vi "Unpack Package.vi"(6 "Overwrite Target Directory if exists (TRUE)?":bool=TRUE, 8 "error in (no error)":errorcluster, 10 "Target directory (same as Package file if empty)":path, 11 "Package File":path) -> (0 "error out":errorcluster, 2 "Unpacked files":path[](array[path]), 3 "Unpacked Package Directory":path)   [LabVIEW 2020]
uses:
  <vilib>/zip/NI_Unzip.lvlib
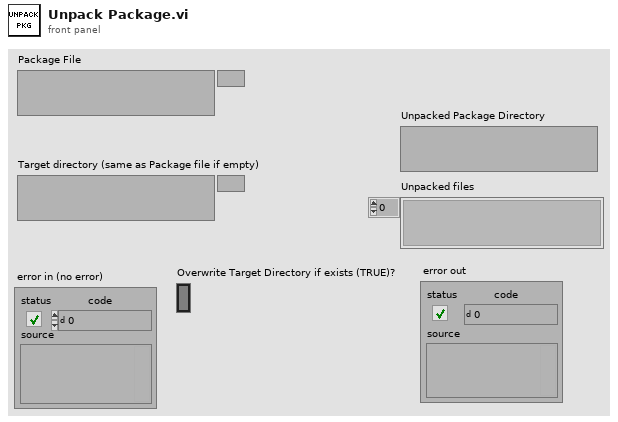
[diagram p1: front panel]
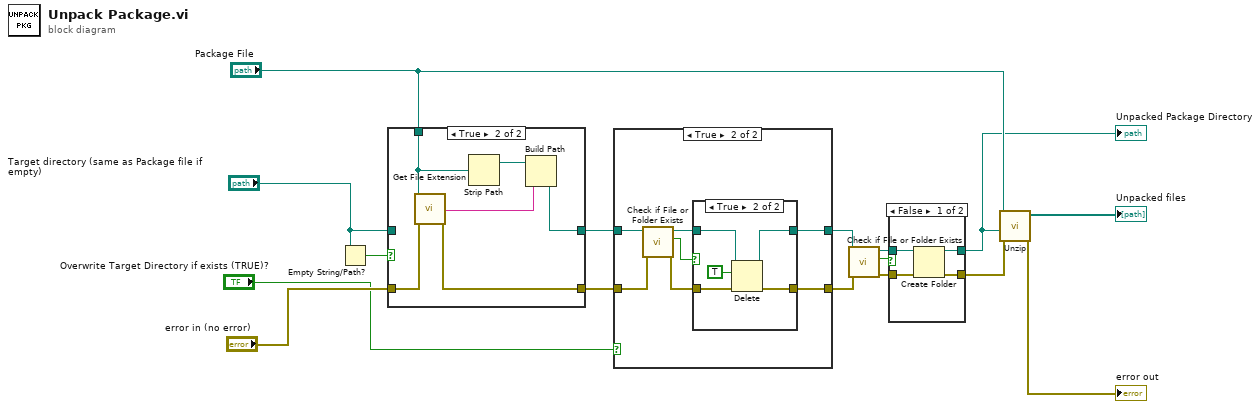
[diagram p0: block diagram]
diagram:
  n1 = Empty String/Path?(string/path="Target directory (same as Package file if empty)") -> (empty?=w16:bool)
  n2 = case shown="True" w16 {
    tunnel: "Package File" -> [_ w22]
    tunnel: "error in (no error)" -> [w18 w21]
    tunnel: [w18 w20] -> w13
    tunnel: [w17 w19] -> w12
    tunnel: "Target directory (same as Package file if empty)" -> [w17 _]
    frame False {
    }
    frame True {
      n3 = call <vilib>:"Get File Extension.vi"("error in (no error)"=w21, "file"=w22) -> ("error out"=w20:errorcluster, "filename without extension"=w23:string)  [unwired: 5 in, 3 out]
      n4 = Strip Path(path=w22) -> (stripped path=w24:path)  [unwired: 1 out]
      n5 = Build Path(base path=w24, name or relative path=w23) -> (appended path=w19:path)
    }
  }
  n6 = case shown="True" "Overwrite Target Directory if exists (TRUE)?" {
    tunnel: w13 -> [w25 w33]
    tunnel: w12 -> [w26 w32]
    tunnel: [w26 w28] -> w5
    tunnel: [w25 w27] -> w4
    frame False {
    }
    frame True {
      n7 = call <vilib>:"Check if File or Folder Exists.vi"("error in (no error)"=w33, "path"=w32) -> ("error out"=w30:errorcluster, "file or folder exists?"=w31:bool, "dup path"=w29:path)  [unwired: 7 in]
      n8 = case shown="True" w31 {
        tunnel: w30 -> [w35 w40]
        tunnel: w29 -> [w34 w38]
        tunnel: [w34 w37] -> w28
        tunnel: [w35 w36] -> w27
        frame False {
        }
        frame True {
          n9 = Delete(path (use dialog)=w38, entire hierarchy (F)=TRUE, error in=w40) -> (deleted path=w37:path, error out=w36:errorcluster)  [unwired: 2 in, 1 out]
        }
      }
    }
  }
  n10 = call <vilib>:"Check if File or Folder Exists.vi"("error in (no error)"=w4, "path"=w5) -> ("error out"=w7:errorcluster, "file or folder exists?"=w1:bool, "dup path"=w6:path)  [unwired: 7 in]
  n11 = case shown="False" w1 {
    tunnel: w7 -> [w44 w45]
    tunnel: w6 -> [w43 w46]
    tunnel: [w42 w46] -> w3
    tunnel: [w41 w45] -> w2
    frame False {
      n12 = Create Folder(path (use dialog)=w43, error in=w44) -> (created path=w42:path, error out=w41:errorcluster)  [unwired: 1 in, 1 out]
    }
    frame True {
    }
  }
  "Unpacked Package Directory" <- w3
  n13 = call <vilib>:"Unzip.vi"("error in (no error)"=w2, "Target directory (same as Zip file if empty)"=w3, "Zip file"="Package File") -> ("error out"=→"error out":errorcluster, "Unzipped files"=→"Unpacked files":path[])  [unwired: 6 in, 1 out]
